vi "ExSubNframesetup.vi"(0 "Camera Handle":u32, 1 "Timing Mode":u32=3 min=1 max=6 step=1, 2 "Intensifier":bool, 3 "error in (no error)":errorcluster, 4 "Exposure":dbl min=0.0 step=0.001 format="%.3f", 5 "Trigger Edge":u32=1 min=1 max=2 step=1, 8 "Number of Images":u32=1 min=1 step=1) -> (6 "Camera handle":u32, 10 "error out":errorcluster)   [LabVIEW 2010]
panel:
  # "Still cleaning this up, name will change in future"
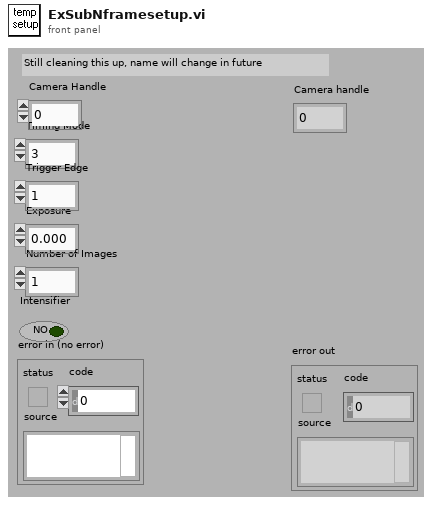
[diagram p1: front panel]
types:
  T1 = cluster{"acquire focus mode":u32, "Exposure":dbl, "Number of Images":u32, "Software accumulation":u32}
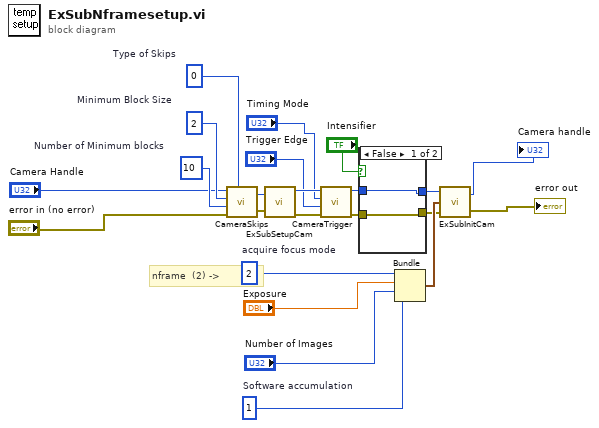
[diagram p0: block diagram]
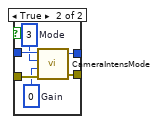
[diagram p2: hidden frame]
diagram:
  w14 = u32 2  # acquire focus mode
  w13 = u32 1  # Software accumulation
  w15 = u32 0  # Type of Skips
  w16 = u32 2  # Minimum Block Size
  w17 = u32 10  # Number of Minimum blocks
  # "nframe  (2) ->"
  n1 = call <userlib>:"CameraSkips.vi"("Camera Handle"="Camera Handle", "Minimum Block Size"=w16, "Number of Minimum blocks"=w17, "error in"="error in (no error)", "Type of Skips"=w15) -> ("Camera Handle"=w19:u32, "error out"=w18:errorcluster)
  n2 = call "ExSubSetupCam.vi"("error in (no error)"=w18, "Camera Handle"=w19) -> ("error out"=w20:errorcluster, "Camera Handle"=w21:u32)
  n3 = call <userlib>:"CameraTrigger.vi"("error in"=w20, "Trigger Edge"="Trigger Edge", "Timing Mode"="Timing Mode", "Camera Handle"=w21) -> ("error out"=w10:errorcluster, "Camera Handle"=w12:u32)
  n4 = case shown="False" "Intensifier" {
    tunnel: w12 -> [w25 w31]
    tunnel: [w25 w30] -> w11
    tunnel: w10 -> [w24 w29]
    tunnel: [w24 w28] -> w9
    frame False {
    }
    frame True {
      w26 = u32 0  # Gain
      w27 = u32 3  # Mode
      n5 = call <userlib>:"CameraIntensMode.vi"("error in"=w29, "Intensifier Gain"=w26, "Mode"=w27, "Camera Handle"=w31) -> ("error out"=w28:errorcluster, "Camera Handle"=w30:u32)
    }
  }
  n6 = Bundle("acquire focus mode"=w14, "Exposure"="Exposure", "Number of Images"="Number of Images", "Software accumulation"=w13) -> (w22:T1)  [unwired: 1 in]
  n7 = call "ExSubInitCam.vi"("error in (no error)"=w9, "Camera Information"=w22, "Camera Handle"=w11) -> ("error out"=→"error out":errorcluster, "Camera Handle"=→"Camera handle":u32)
